vi "Ticks per decisecond to Feet per second.vi"(11 "Drive Velocities (ticks/ds)":T1) -> (3 "Drive Velocities (ft/s)":T1)   [LabVIEW 2020]
doc: "converts ticks per decisecond (falcon units) to feet per second"
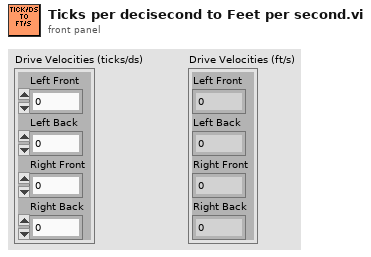
[diagram p1: front panel]
types:
  T1 = cluster{"Left Front":i32, "Left Back":i32, "Right Front":i32, "Right Back":i32}
  T2 = cluster{"Left Front":dbl, "Left Back":dbl, "Right Front":dbl, "Right Back":dbl}
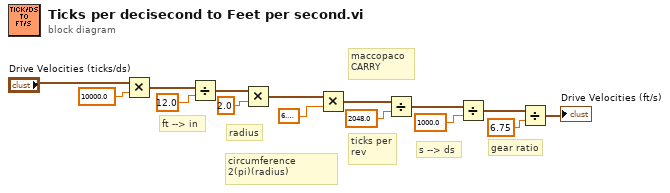
[diagram p0: block diagram]
diagram:
  # "s --> ds"
  # "circumference\n2(pi)(radius)"
  # "ticks per\nrev"
  # "ft --> in"
  # "radius"
  # "gear ratio"
  # "maccopaco\nCARRY"
  n1 = Multiply(x="Drive Velocities (ticks/ds)", y=10000.0) -> (x*y=w14:T2)
  n2 = Divide(x=w14, y=12.0) -> (x/y=w12:T2)
  n3 = Multiply(x=w12, y=2.0) -> (x*y=w10:T2)
  n4 = Multiply(x=w10, y=6.283185307179586) -> (x*y=w9:T2)
  n5 = Divide(x=w9, y=2048.0) -> (x/y=w7:T2)
  n6 = Divide(x=w7, y=1000.0) -> (x/y=w5:T2)
  n7 = Divide(x=w5, y=6.75) -> (x/y=→"Drive Velocities (ft/s)":T2)
